vi "Format DF1-DF2.vi"(10 "Resutls In":T1) -> (2 "Results Out":T1)   [LabVIEW 2015, in "niDTS BT.lvlib" / "niDTS BT INSTR TX.lvclass"]
uses:
  niDTS BT INSTR TX.lvclass
  Includes/niDTS BT INSTR TX INC ModAcc Result.ctl
  Tests/Tx Test/Includes/niDTS BT Tx Test INC DEVM Results.ctl
  Tests/Tx Test/Includes/niDTS BT Tx Test INC CF Stability Results.ctl
  Tests/Tx Test/Includes/niDTS BT Tx Test INC CFO Resutls.ctl
  Tests/Tx Test/Includes/niDTS BT Tx Test INC Character Results.ctl
  niDTS BT.lvlib
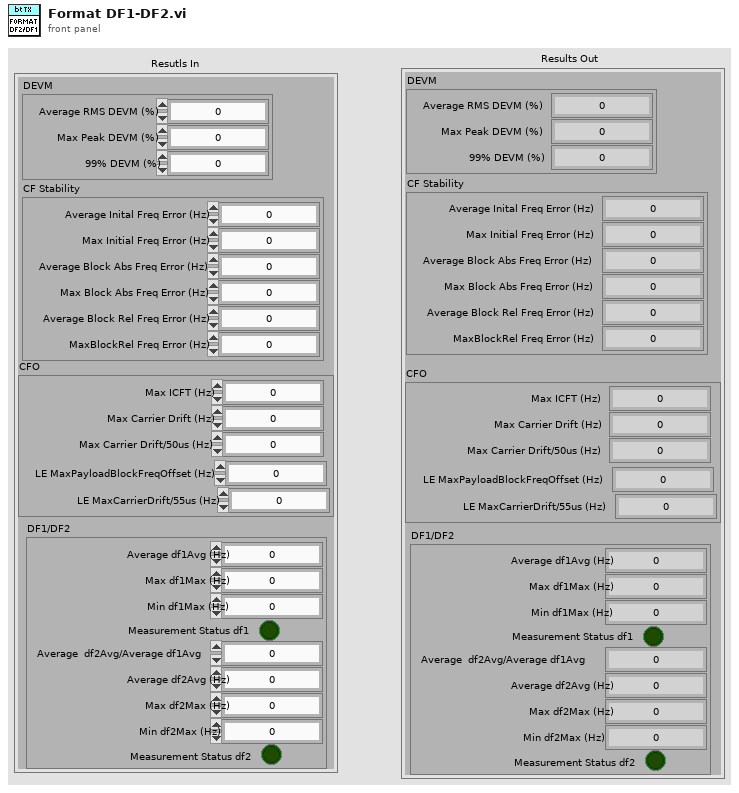
[diagram p1: front panel]
types:
  T1 = typedef "niDTS BT.lvlib/niDTS BT INSTR TX.lvclass/niDTS BT INSTR TX INC ModAcc Result.ctl" = cluster{"DEVM":T2, "CF Stability":T3, "CFO":T4, "DF1/DF2":T5}
  T2 = typedef "niDTS BT.lvlib/niDTS BT Tx Test INC DEVM Results.ctl" = cluster{"Average RMS DEVM (%)":dbl, "Max Peak DEVM (%)":dbl, "99% DEVM (%)":dbl}
  T3 = typedef "niDTS BT.lvlib/niDTS BT Tx Test INC CF Stability Results.ctl" = cluster{"Average Inital Freq Error (Hz)":dbl, "Max Initial Freq Error (Hz)":dbl, "Average Block Abs Freq Error (Hz)":dbl, "Max Block Abs Freq Error (Hz)":dbl, "Average Block Rel Freq Error (Hz)":dbl, "MaxBlockRel Freq Error (Hz)":dbl}
  T4 = typedef "niDTS BT.lvlib/niDTS BT Tx Test INC CFO Resutls.ctl" = cluster{"Max ICFT (Hz)":dbl, "Max Carrier Drift (Hz)":dbl, "Max Carrier Drift/50us (Hz)":dbl, "LE MaxPayloadBlockFreqOffset (Hz)":dbl, "LE MaxCarrierDrift/55us (Hz)":dbl}
  T5 = typedef "niDTS BT.lvlib/niDTS BT Tx Test INC Character Results.ctl" = cluster{"Average df1Avg (Hz)":dbl, "Max df1Max (Hz)":dbl, "Min df1Max (Hz)":dbl, "Measurement Status df1":bool, "Average  df2Avg/Average df1Avg":dbl, "Average df2Avg (Hz)":dbl, "Max df2Max (Hz)":dbl, "Min df2Max (Hz)":dbl, "Measurement Status df2":bool}
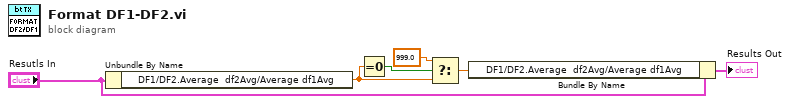
[diagram p0: block diagram]
diagram:
  n1 = Unbundle By Name("Resutls In") -> ("DF1/DF2.Average  df2Avg/Average df1Avg"=w1:dbl)
  n2 = Equal To 0?(x=w1) -> (x = 0?=w6:bool)
  n3 = Select(t=999.0, s=w6, f=w1) -> (s? t:f=w4:dbl)
  n4 = Bundle By Name(cluster="Resutls In", "DF1/DF2.Average  df2Avg/Average df1Avg"=w4) -> (→"Results Out":T1)
